vi "FRCts20_Backend_INI_Increment_Build_Number.vi"   [LabVIEW 2014, in "FRCts20_Backend_Engine.lvlib" / "FRCts20_Backend_INI Controller.lvclass"]
uses:
  FRCts20_Backend_INI Controller.lvclass
  FRCts20_Backend_Engine.lvlib
types:
  T1 = typedef "FRCts20_Backend_Engine.lvlib/FRCts20_Backend_INI Controller.lvclass/FRCts20_Backend_INI_Revision.ctl" = cluster{"Major Revision":i32, "Minor Revision":i32, "Branch Number":i32, "Build Phase":string, "Build Number":i32}
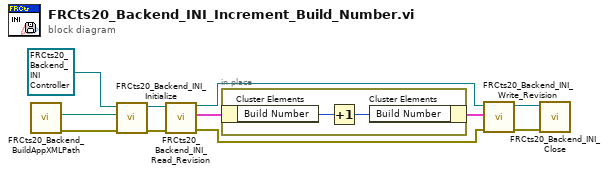
[diagram p0: block diagram]
diagram:
  n1 = call "FRCts20_Backend_BuildAppXMLPath.vi"() -> ("error out"=w10:errorcluster, "Path Out"=w9:path)  [unwired: 10 in]
  n2 = call "FRCts20_Backend_INI_Initialize.vi"("error in (no error)"=w10, "Config Path"=w9, "INI Controller in"=refnum<class "FRCts20_Backend_INI Controller.lvclass"> refnum ("FRCts20_Backend_Engine.lvlib:INI Controller.lvclass")) -> ("error out"=w8:errorcluster, "INI Controller out"=w7:refnum<class "FRCts20_Backend_INI Controller.lvclass">)  [unwired: 7 in]
  n3 = call "FRCts20_Backend_INI_Read_Revision.vi"("error in (no error)"=w8, "INI Controller in"=w7) -> ("error out"=w3:errorcluster, "Revision"=w6:T1, "INI Controller out"=w4:refnum<class "FRCts20_Backend_INI Controller.lvclass">)  [unwired: 7 in]
  n4 = in-place {
    n5 = in-place-cluster #1(w6) -> ("Build Number"=w12:i32)
    n6 = Increment(x=w12) -> (x+1=w13:i32)
    n7 = in-place-cluster #1("Build Number"=w13) -> (w5:T1)
  }
  n8 = call "FRCts20_Backend_INI_Write_Revision.vi"("error in (no error)"=w3, "Revision"=w5, "INI Controller in"=w4) -> ("error out"=w1:errorcluster, "INI Controller out"=w2:refnum<class "FRCts20_Backend_INI Controller.lvclass">)  [unwired: 7 in]
  n9 = call "FRCts20_Backend_INI_Close.vi"("error in (no error)"=w1, "INI Controller in"=w2) -> ()  [unwired: 7 in, 3 out]
